vi "FGVBackgroundORT.vi"(6 "Corrected...In":bool, 7 "Enum":T1, 8 "error in":errorcluster, 9 "arrayIn":i16[](array[numeric]), 10 "Wave In":dbl[](array[numeric]), 11 "Wave In Shifted":dbl[](array[numeric])) -> (0 "error out":errorcluster, 1 "arrayOut":i16[](array[numeric]), 2 "Wave Out":dbl[](array[numeric]), 3 "Wave Out Shifted":dbl[](array[numeric]), 4 "Corrected...Out":bool)   [LabVIEW 2016]
uses:
  controls/Enum.ctl
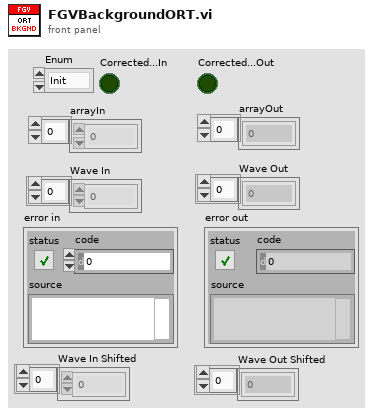
[diagram p1: front panel]
types:
  T1 = typedef "Enum.ctl" = enum16{"Init", "Read", "Write"}
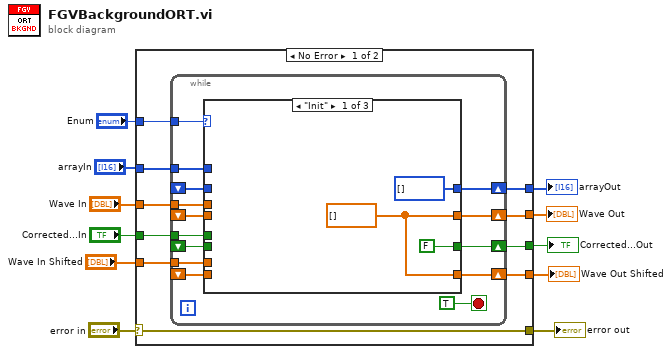
[diagram p0: block diagram]
diagram:
  n1 = case shown="No Error" "error in" {
    selector: "error in" -> [w20 w51]
    tunnel: "Enum" -> [w21 _]
    tunnel: [w20 w51] -> w10
    tunnel: "arrayIn" -> [w19 w50]
    tunnel: [w18 w50] -> w8
    tunnel: "Wave In" -> [w17 w49]
    tunnel: [w16 w49] -> w5
    tunnel: "Corrected...In" -> [w15 w48]
    tunnel: [w14 w48] -> w3
    tunnel: [w12 w47] -> w2
    tunnel: "Wave In Shifted" -> [w13 w47]
    frame No Error {
      n2 = while {
        tunnel: w21 -> [w34]
        tunnel: w19 -> [w33]
        shift-right: [w32] -> w18
        shift-left: _ -> [w31]
        tunnel: w17 -> [w30]
        shift-right: [w29] -> w16
        shift-left: _ -> [w28]
        tunnel: w15 -> [w27]
        shift-right: [w26] -> w14
        shift-left: _ -> [w25]
        tunnel: w13 -> [w22]
        shift-right: [w24] -> w12
        shift-left: _ -> [w23]
        stop <- TRUE stop-if-true
        n3 = case shown="\"Init\"" w34 {
          tunnel: w33 -> [_ _ w46]
          tunnel: [i16[] [] ("arrayIn") w42 w46] -> w32
          tunnel: w31 -> [_ w42 _]
          tunnel: w30 -> [_ _ w45]
          tunnel: [w36 w41 w45] -> w29
          tunnel: w28 -> [_ w41 _]
          tunnel: w27 -> [_ _ w44]
          tunnel: [FALSE ("Corrected...In") w40 w44] -> w26
          tunnel: w25 -> [_ w40 _]
          tunnel: w23 -> [_ w39 _]
          tunnel: [w36 w39 w43] -> w24
          tunnel: w22 -> [_ _ w43]
          frame "Init" {
            w36 = dbl[] [] ("Wave In")
          }
          frame "Read", Default {
          }
          frame "Write" {
          }
        }
      }
    }
    frame Error {
    }
  }
  "error out" <- w10
  "arrayOut" <- w8
  "Wave Out" <- w5
  "Corrected...Out" <- w3
  "Wave Out Shifted" <- w2
